vi "PowerSlideGetSetRefNum.vi"(8 "error in (no error)":errorcluster, 9 "menu":T11, 10 "refnum name":string, 11 "PowerSlideDevRef":T10) -> (0 "error out":errorcluster, 2 "names":string[](array[string]), 3 "PowerSlideDevRef 2":T10)   [LabVIEW 2014, in "PowerSlide.lvlib"]
doc: "Sets a reference into a registry, gets a reference from a registry, or deletes a reference from a registry. The reference is accessed by name, and can be given any unique name.\n\nThis software is licensed. Open the labview\\readme\\WPI Robotics Library Open Source License.txt file for more information."
uses:
  PowerSlide.lvlib
  <vilib>/Rock Robotics/WPI/Utilities/Refnum Registry Operation.ctl
  <vilib>/Rock Robotics/WPI/MotorControl/WPI_MotorControlDeviceRef.ctl
  <vilib>/Rock Robotics/WPI/MotorControl/WPI_MotorControlType.ctl
  <vilib>/Rock Robotics/SystemInterfaces/Typedef/FPGA_TypedefDigitalModule.ctl
  <vilib>/Rock Robotics/SystemInterfaces/DIO/FPGA_DIOPWMChannel.ctl
  <vilib>/Rock Robotics/WPI/PWM/WPI_PWMDeadband.ctl
  <vilib>/Rock Robotics/WPI/CAN/Jaguar/SubVIs/WPI_CANJaguar_ControlMode.ctl
  <vilib>/Rock Robotics/WPI/CAN/TalonSRX/WPI_CANTalonSRX_APIControlMode.ctl
  <vilib>/Rock Robotics/WPI/PWM/WPI_PWMTransform_ConPane.ctl
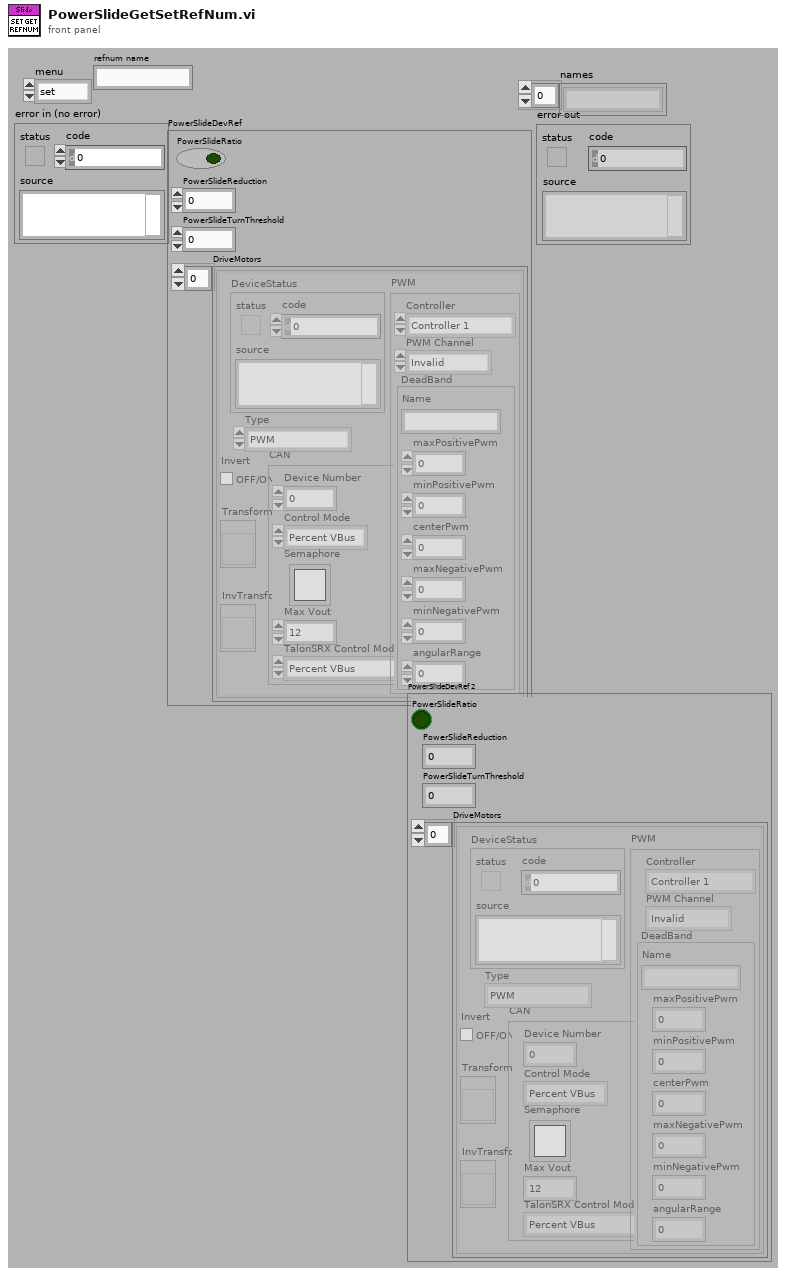
[diagram p1: front panel]
types:
  T1 = typedef "WPI_MotorControlDeviceRef.ctl" = cluster{"DeviceStatus":errorcluster, "Type":T2, "PWM":cluster{"Controller":T3, "PWM Channel":T4, "DeadBand":T5}, "CAN":cluster{"Device Number":u8, "Control Mode":T6, "Semaphore":T7, "Max Vout":dbl, "TalonSRX Control Mode":T8}, "Invert":bool, "TransformRef":T9, "InvTransformRef":T9}
  T2 = typedef "WPI_MotorControlType.ctl" = enum16{"PWM", "CAN", "CANTalonSRX"}
  T3 = typedef "FPGA_TypedefDigitalModule.ctl" = enum16{"Controller 1"}
  T4 = typedef "FPGA_DIOPWMChannel.ctl" = enum8{"PWM 0", "PWM 1", "PWM 2", "PWM 3", "PWM 4", "PWM 5", "PWM 6", "PWM 7", "PWM 8", "PWM 9", "PWM MXP 0", "PWM MXP 1", "PWM MXP 2", "PWM MXP 3", "PWM MXP 4", "PWM MXP 5", "PWM MXP 6", "PWM MXP 7", "PWM MXP 8", "PWM MXP 9", "Invalid"}
  T5 = typedef "WPI_PWMDeadband.ctl" = cluster{"Name":string, "maxPositivePwm":i32, "minPositivePwm":i32, "centerPwm":i32, "maxNegativePwm":i32, "minNegativePwm":i32, "angularRange":u16}
  T6 = typedef "WPI_CANJaguar_ControlMode.ctl" = enum8{"Percent VBus", "Current", "Speed", "Position", "Voltage"}
  T7 = typedef "Semaphore RefNum" = refnum<k1>
  T8 = typedef "WPI_CANTalonSRX_APIControlMode.ctl" = enum8{"Percent VBus", "Speed", "Position", "Slave", "Unchanged / Invalid"}
  T9 = typedef "WPI_PWMTransform_ConPane.ctl" = refnum<vi>
  T10 = cluster{"PowerSlideRatio":bool, "PowerSlideReduction":dbl, "PowerSlideTurnThreshold":dbl, "DriveMotors":T1[]}
  T11 = typedef "Refnum Registry Operation.ctl" = enum16{"set", "get", "delete", "get all names", "read name"}
  T12 = cluster{"PowerSlideRatio":bool, "PowerSlideReduction":dbl, "PowerSlideTurnThreshold":dbl, "DriveMotors":T1[]}[]
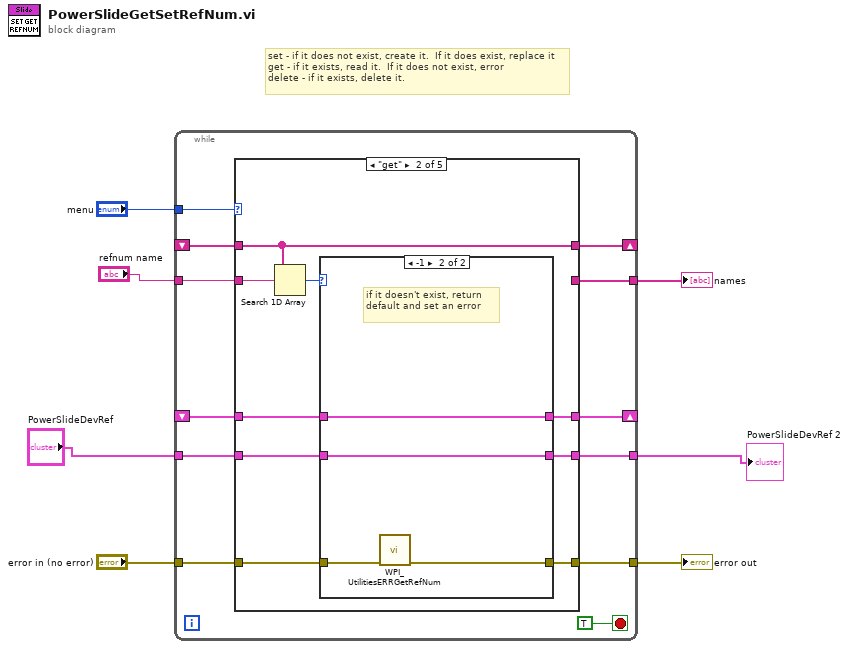
[diagram p0: block diagram]
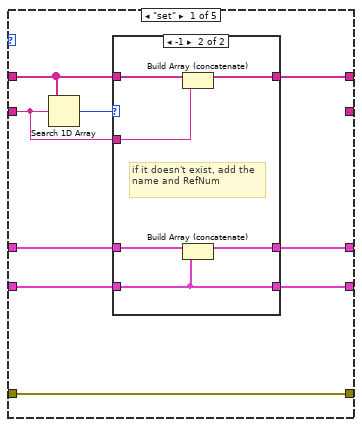
[diagram p2: hidden frame]
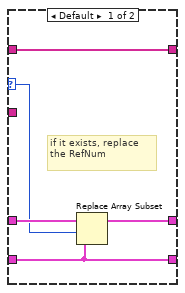
[diagram p3: hidden frame]
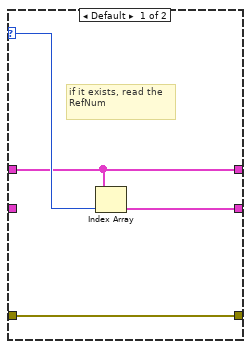
[diagram p4: hidden frame]
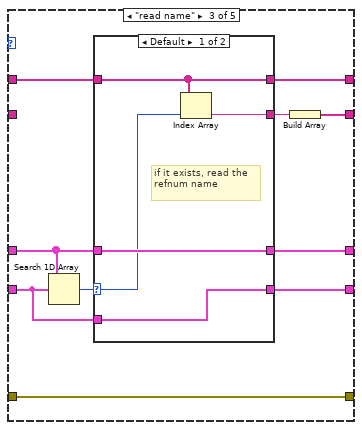
[diagram p5: hidden frame]
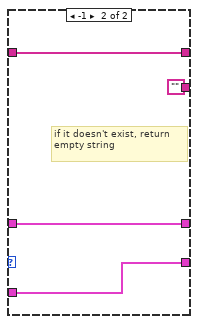
[diagram p6: hidden frame]
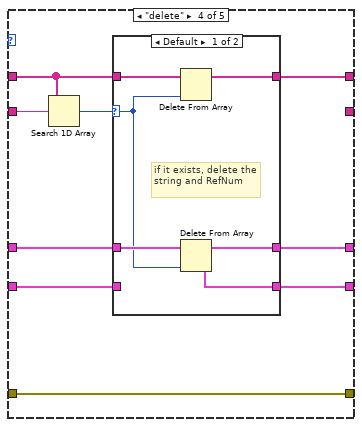
[diagram p7: hidden frame]
diagram:
  # "set - if it does not exist, create it.  If it does exist, replace it\nget - if it exists, read it.  If it does not exist, error\ndelete - if it exists, delete it."
  n1 = while {
    tunnel: "PowerSlideDevRef" -> [w19]
    tunnel: "refnum name" -> [w12]
    tunnel: "error in (no error)" -> [w11]
    shift-right: [w18] -> _
    shift-left: _ -> [w17]
    tunnel: [w16] -> w1
    tunnel: "menu" -> [w15]
    shift-right: [w14] -> _
    shift-left: _ -> [w13]
    tunnel: [w10] -> w6
    tunnel: [w8] -> w4
    stop <- TRUE stop-if-true
    n2 = case shown="\"get\"" w15 {
      tunnel: w19 -> [w23 w46 w58 w80 w95]
      tunnel: [w22 w45 w66 w79 w96] -> w18
      tunnel: w17 -> [w24 w47 w64 w81 w96]
      tunnel: [w21 w44 w65 w78 w95] -> w16
      tunnel: [w28 w43 w60 w84 w97] -> w14
      tunnel: w13 -> [w27 w43 w61 w83 w97]
      tunnel: w12 -> [w25 w40 _ w76 _]
      tunnel: [w20 w41 w62 w77 w94] -> w10
      tunnel: w11 -> [w20 w42 w62 w77 w94]
      tunnel: [_ _ w57 _ w97] -> w8
      frame "set" {
        n3 = Search 1D Array(1D array=w27, element=w25) -> (index of element=w26:i32)  [unwired: 1 out]
        n4 = case shown="-1" w26 {
          selector: w26 -> [w31 _]
          tunnel: [w33 w39] -> w28
          tunnel: w27 -> [w33 w38]
          tunnel: w25 -> [_ w34]
          tunnel: w24 -> [w32 w37]
          tunnel: w23 -> [w29 w35]
          tunnel: [w30 w36] -> w22
          tunnel: [w29 w35] -> w21
          frame Default {
            # "if it exists, replace the RefNum"
            n5 = Replace Array Subset(array=w32, new element=w29, index=w31) -> (w30:T12)
          }
          frame -1 {
            # "if it doesn't exist, add the name and RefNum"
            n6 = Build Array (concatenate)(w38, w34) -> (w39:string[])
            n7 = Build Array (concatenate)(w37, w35) -> (w36:T12)
          }
        }
      }
      frame "get" {
        n8 = Search 1D Array(1D array=w43, element=w40) -> (index of element=w48:i32)  [unwired: 1 out]
        n9 = case shown="-1" w48 {
          selector: w48 -> [w52 _]
          tunnel: w47 -> [w50 w56]
          tunnel: w46 -> [_ w53]
          tunnel: [w50 w56] -> w45
          tunnel: [w51 w53] -> w44
          tunnel: w42 -> [w49 w55]
          tunnel: [w49 w54] -> w41
          frame Default {
            # "if it exists, read the RefNum"
            n10 = Index Array(array=w50, index=w52) -> (element=w51:T10)
          }
          frame -1 {
            # "if it doesn't exist, return default and set an error"
            n11 = call <vilib>:"WPI_UtilitiesERRGetRefNum.vi"("error in (no error)"=w55) -> ("ERRGetRefNum"=w54:errorcluster)  [unwired: 10 out]
          }
        }
      }
      frame "read name" {
        n12 = Search 1D Array(1D array=w64, element=w58) -> (index of element=w63:i32)  [unwired: 1 out]
        n13 = case shown="Default" w63 {
          selector: w63 -> [w68 _]
          tunnel: w64 -> [w71 w75]
          tunnel: [w71 w75] -> w66
          tunnel: [w67 w74] -> w65
          tunnel: w61 -> [w69 w73]
          tunnel: [w69 w73] -> w60
          tunnel: [w70 ""] -> w59
          tunnel: w58 -> [w67 w74]
          frame Default {
            # "if it exists, read the refnum name"
            n14 = Index Array(array=w69, index=w68) -> (element=w70:string)
          }
          frame -1 {
            # "if it doesn't exist, return empty string"
          }
        }
        n15 = Build Array(w59) -> (w57:string[])
      }
      frame "delete" {
        n16 = Search 1D Array(1D array=w83, element=w76) -> (index of element=w82:i32)  [unwired: 1 out]
        n17 = case shown="Default" w82 {
          selector: w82 -> [w85 _]
          tunnel: [w86 w92] -> w84
          tunnel: w83 -> [w87 w92]
          tunnel: w81 -> [w90 w91]
          tunnel: w80 -> [_ w93]
          tunnel: [w89 w91] -> w79
          tunnel: [w88 w93] -> w78
          frame Default {
            # "if it exists, delete the string and RefNum"
            n18 = Delete From Array(array=w87, index=w85) -> (array with subset deleted=w86:string[])  [unwired: 1 in, 1 out]
            n19 = Delete From Array(array=w90, index=w85) -> (deleted portion=w88:T10, array with subset deleted=w89:T12)  [unwired: 1 in]
          }
          frame -1 {
            # "if it doesn't exist, do nothing"
          }
        }
      }
      frame "get all names", Default {
      }
    }
  }
  "error out" <- w6
  "names" <- w4
  "PowerSlideDevRef 2" <- w1
